vi "CU_CohenKappa.vi"(4 "Confusion Matrix":i32[][](array[numeric])) -> (1 "CohenKappa":dbl)   [LabVIEW 2016, in "Classifier.lvlib"]
uses:
  Classifier.lvlib
panel:
  # "This VI is a part of BCI Design library, http://www.ru-bci.org \nCopyright © 2020, Sotnikov Peter, All rights reserved. License: GNU GPLv3"
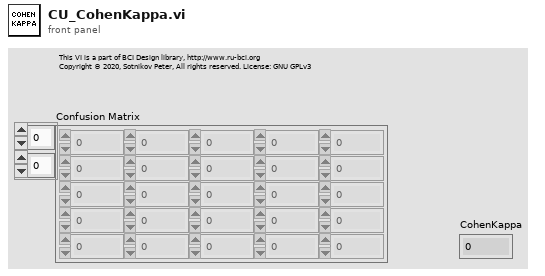
[diagram p1: front panel]
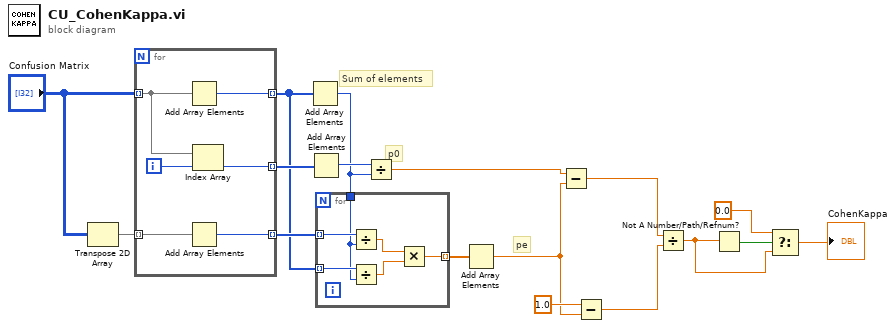
[diagram p0: block diagram]
diagram:
  # "Sum of elements"
  # "pe"
  # "p0"
  n1 = Transpose 2D Array(2D array="Confusion Matrix") -> (transposed array=w15:i32[][])
  n2 = for {
    tunnel: "Confusion Matrix" -> [w22] mode=indexing
    tunnel: [w23] -> w12 mode=indexing
    tunnel: w15 -> [w19] mode=indexing
    tunnel: [w20] -> w14 mode=indexing
    tunnel: [w18] -> w13 mode=indexing
    i -> [w21]
    n3 = Add Array Elements(numeric array=w22) -> (sum=w23:i32)
    n4 = Add Array Elements(numeric array=w19) -> (sum=w18:i32)
    n5 = Index Array(array=w22, index=w21) -> (element=w20:i32)
  }
  n6 = Add Array Elements(numeric array=w12) -> (sum=w5:i32)
  n7 = Add Array Elements(numeric array=w14) -> (sum=w16:i32)
  n8 = for {
    tunnel: w13 -> [w28] mode=indexing
    tunnel: w12 -> [w26] mode=indexing
    tunnel: [w29] -> w10 mode=indexing
    tunnel: w5 -> [w24]
    n9 = Divide(x=w28, y=w24) -> (x/y=w27:dbl)
    n10 = Divide(x=w26, y=w24) -> (x/y=w25:dbl)
    n11 = Multiply(x=w27, y=w25) -> (x*y=w29:dbl)
  }
  n12 = Divide(x=w16, y=w5) -> (x/y=w11:dbl)
  n13 = Add Array Elements(numeric array=w10) -> (sum=w6:dbl)
  n14 = Subtract(x=w11, y=w6) -> (x-y=w8:dbl)
  n15 = Subtract(x=1.0, y=w6) -> (x-y=w7:dbl)
  n16 = Divide(x=w8, y=w7) -> (x/y=w3:dbl)
  n17 = Not A Number/Path/Refnum?(number/path/refnum=w3) -> (NaN/Path/Refnum?=w4:bool)
  n18 = Select(t=0.0, s=w4, f=w3) -> (s? t:f=→"CohenKappa":dbl)
